vi "Initialize frame array.vi"(11 "Buffer size":i32) -> (3 "Frame buffer":T1[](array[typedef]))   [LabVIEW 2018]
uses:
  <vilib>/vision/Image Controls.llb/IMAQ Image.ctl
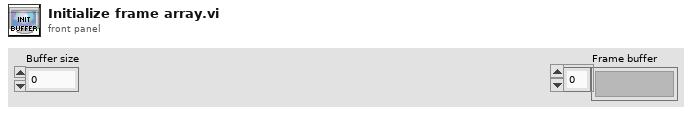
[diagram p1: front panel]
types:
  T1 = typedef "IMAQ Image.ctl" = refnum<image>
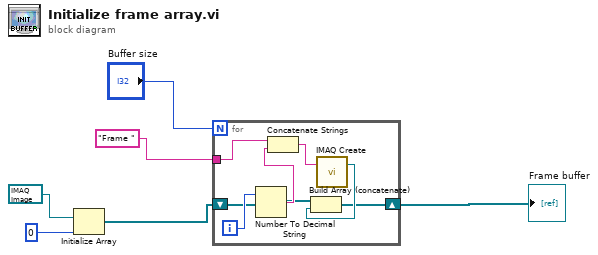
[diagram p0: block diagram]
diagram:
  n1 = Initialize Array(T1 refnum ("New Image"), 0) -> (w4:T1[])
  n2 = for {
    N: "Buffer size" -> [_]
    tunnel: "Frame " ("Image Name") -> [w13]
    shift-right: [w7] -> w2
    shift-left: w4 -> [w8]
    i -> [w12]
    n3 = Number To Decimal String(number=w12) -> (decimal integer string=w11:string)  [unwired: 1 in]
    n4 = Concatenate Strings(w13, w11) -> (w10:string)
    n5 = call "IMAQ Create"("Image Name"=w10) -> ("New Image"=w9:T1)  [unwired: 4 in, 1 out]
    n6 = Build Array (concatenate)(w8, w9) -> (w7:T1[])
  }
  "Frame buffer" <- w2
